vi "RSZVB Set Time Domain Transformation Filter.vi"(8 "error in (no error)":errorcluster {"code" format="%.0x"}, 9 "Filter Type (0: No profiling (rectangle))":i32(ring) items=["No profiling (rectangle)", "Normal profile (Hann)", "Low first sidelobe (Hamming)", "Steep falloff (Bohman)", "Arbitrary sidelobes (Dolph-Chebychev)"], 10 "Channel (Trace) (1)":i32=1, 11 "VISA session":refnum<visa-resource-name>) -> (0 "error out":errorcluster {"code" format="%.0x"}, 3 "dup VISA session":refnum<visa-resource-name>)   [LabVIEW 2011]
doc: "This VI selects the window type for filtering the data in the frequency domain prior to the time domain transformation.\n\nRemote-control command(s):\nCALCulate<Ch/Tr>:TRANsform:TIME:WINDow RECT | HAMMing | HANN | BOHMan | DCHebyshev"
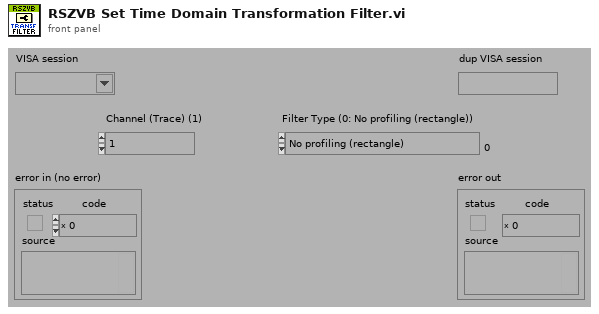
[diagram p1: front panel]
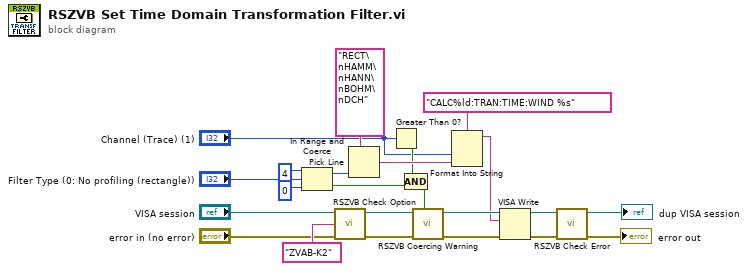
[diagram p0: block diagram]
diagram:
  n1 = In Range and Coerce(upper limit=4, x="Filter Type (0: No profiling (rectangle))", lower limit=0) -> (coerced(x)=w10:i32, In Range?=w13:bool)
  n2 = call "RSZVB Check Option.vi"("error in (no error)"="error in (no error)", "Options"="ZVAB-K2", "VISA session"="VISA session") -> ("error out"=w9:errorcluster, "dup VISA session"=w8:refnum<visa-resource-name>)  [unwired: 7 in]
  n3 = Pick Line(multi-line string="RECT\nHAMM\nHANN\nBOHM\nDCH", line index=w10) -> (output string=w16:string)  [unwired: 1 in]
  n4 = Greater Than 0?(x="Channel (Trace) (1)") -> (x > 0?=w12:bool)
  n5 = Compound Arithmetic op=AND(w12, w13) -> (w11:bool)
  n6 = call "RSZVB Coercing Warning.vi"("In Range?"=w11, "error in (no error)"=w9, "VISA session"=w8) -> ("error out"=w21:errorcluster, "dup VISA session"=w22:refnum<visa-resource-name>)  [unwired: 7 in]
  n7 = Format Into String(format string="CALC%ld:TRAN:TIME:WIND %s", "Channel (Trace) (1)", w16) -> (resulting string=w18:string)  [unwired: 2 in, 1 out]
  n8 = VISA Write(VISA resource name=w22, write buffer=w18, error in (no error)=w21) -> (VISA resource name out=w19:refnum<visa-resource-name>, error out=w20:errorcluster)  [unwired: 1 out]
  n9 = call "RSZVB Check Error.vi"("error in (no error)"=w20, "VISA session"=w19) -> ("error out"=→"error out":errorcluster, "dup VISA session"=→"dup VISA session":refnum<visa-resource-name>)  [unwired: 8 in]
